vi "Clear.vi"(10 "Bit to clear":u8, 11 "Data_In":u16 format="%.0b") -> (3 "Data_Out":u16 format="%.0b")   [LabVIEW 2017, in "Bit Manipulation.lvlib"]
uses:
  Bit Manipulation.lvlib
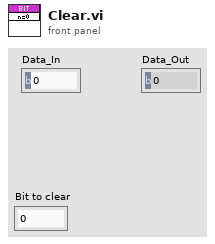
[diagram p1: front panel]
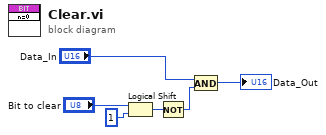
[diagram p0: block diagram]
diagram:
  n1 = Logical Shift(y="Bit to clear", x=u16 1) -> (x << y=w4:u16)
  n2 = Not(x=w4) -> (.not. x?=w3:u16)
  n3 = And(x="Data_In", y=w3) -> (x .and. y?=→"Data_Out":u16)
